vi "Convert_Elapsed_Time_To_Display.vi"(8 "error in (no error)":errorcluster, 11 "Elapsed Time":dbl) -> (0 "error out":errorcluster, 3 "Display Out":string)   [LabVIEW 2026]
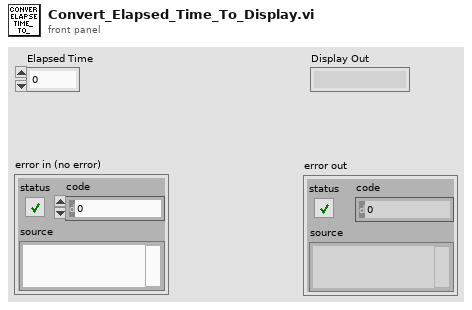
[diagram p1: front panel]
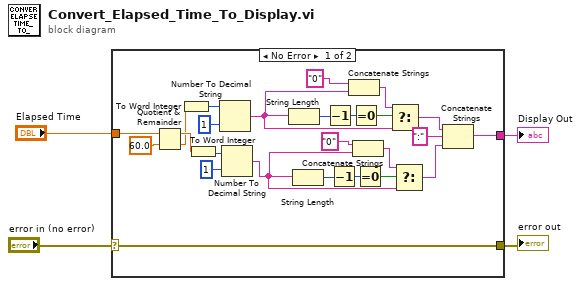
[diagram p0: block diagram]
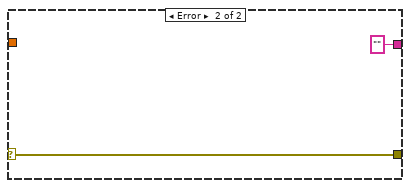
[diagram p2: hidden frame]
diagram:
  n1 = case shown="No Error" "error in (no error)" {
    selector: "error in (no error)" -> [w5 w31]
    tunnel: "Elapsed Time" -> [w29 _]
    tunnel: [w8 ""] -> w3
    tunnel: [w5 w31] -> w1
    frame No Error {
      n2 = Quotient & Remainder(x=w29, y=60.0) -> (x-y*floor(x/y)=w12:dbl, floor(x/y)=w10:dbl)
      n3 = To Word Integer(number=w10) -> (16bit integer=w11:i16)
      n4 = To Word Integer(number=w12) -> (16bit integer=w13:i16)
      n5 = Number To Decimal String(number=w11, width (-)=i16 1 ("precision (6)")) -> (decimal integer string=w20:string)
      n6 = Number To Decimal String(number=w13, width (-)=i16 1) -> (decimal integer string=w26:string)
      n7 = String Length(string=w20) -> (length=w16:i32)
      n8 = String Length(string=w26) -> (length=w23:i32)
      n9 = Decrement(x=w16) -> (x-1=w15:i32)
      n10 = Decrement(x=w23) -> (x-1=w22:i32)
      n11 = Concatenate Strings("0" ("string"), w20) -> (w19:string)
      n12 = Equal To 0?(x=w15) -> (x = 0?=w17:bool)
      n13 = Concatenate Strings("0" ("string"), w26) -> (w25:string)
      n14 = Equal To 0?(x=w22) -> (x = 0?=w24:bool)
      n15 = Select(t=w19, s=w17, f=w20) -> (s? t:f=w21:string)
      n16 = Select(t=w25, s=w24, f=w26) -> (s? t:f=w28:string)
      n17 = Concatenate Strings(w21, ":" ("string"), w28) -> (w8:string)
    }
    frame Error {
    }
  }
  "Display Out" <- w3
  "error out" <- w1
